vi "Read Status Byte Query.vi"(0 "VISA resource name":refnum<visa-resource-name>, 11 "error in (no error)":errorcluster) -> (4 "VISA resource name out":refnum<visa-resource-name>, 6 "Status Byte Register":T1, 15 "error out":errorcluster)   [LabVIEW 2018, in "XP Power PLS600.lvlib"]
doc: "Queries the <B>Status Byte</B>. Returns the decimal value of the binary-weighted sum of bits.\n\nEach bit represents a status in the instrument.\n\nBIT 0: Reserved\nBIT 1: Reserved\nBIT 2: Error in Queue\nBIT 3: QUES = Questionable Status Summary\nBIT 4: MAV = Message Available\nBIT 5: ESB = Event Status Byte Summary\nBIT 6: RQS = Request for Service\nBIT 7: OPER = Operation Event Summary"
uses:
  XP Power PLS600.lvlib
panel:
  # "BIT 0: Reserved\nBIT 1: Reserved\nBIT 2: Error in Queue\nBIT 3: QUES = Questionable Status Summary\nBIT 4: MAV = Message Available\nBIT 5: ESB = Event Status Byte Summary\nBIT 6: RQS = Request for Service\nBIT 7: OPER = Operation Event Summary"
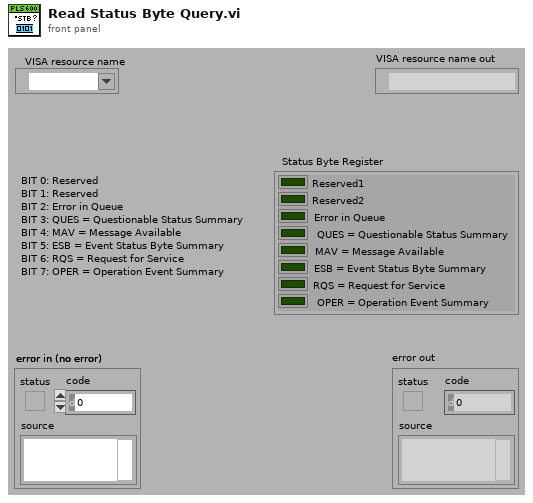
[diagram p1: front panel]
types:
  T1 = cluster{"Reserved1":bool, "Reserved2":bool, "Error in Queue":bool, "QUES = Questionable Status Summary":bool, "MAV = Message Available":bool, "ESB = Event Status Byte Summary":bool, "RQS = Request for Service":bool, "OPER = Operation Event Summary":bool}
  T2 = cluster{"Boolean array[0]":bool, "Boolean array[1]":bool, "Boolean array[2]":bool, "Boolean array[3]":bool, "Boolean array[4]":bool, "Boolean array[5]":bool, "Boolean array[6]":bool, "Boolean array[7]":bool}
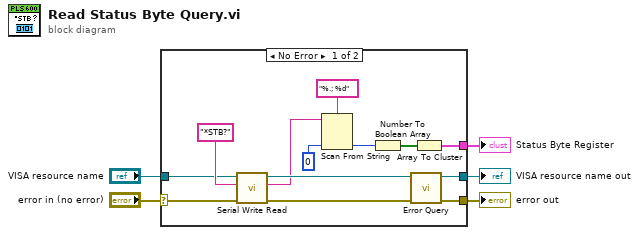
[diagram p0: block diagram]
diagram:
  n1 = case shown="No Error" "error in (no error)" {
    selector: "error in (no error)" -> [w13 w19]
    tunnel: [w18 _] -> w5
    tunnel: "VISA resource name" -> [w12 w20]
    tunnel: [w15 w20] -> w3
    tunnel: [w16 w19] -> w2
    frame No Error {
      n2 = call "Serial Write Read.vi"("error in (no error)"=w13, "Write Buffer"="*STB?" ("Command to Send (empty)"), "VISA resource name"=w12) -> ("error out"=w11:errorcluster, "Read Buffer"=w6:string, "VISA resource name out"=w10:refnum<visa-resource-name>)  [unwired: 6 in]
      n3 = Scan From String(format string="%.; %d" ("Format String"), input string=w6, default 1=u8 0 ("default value 1")) -> (output 1=w7:u8)  [unwired: 2 in, 3 out]
      n4 = Number To Boolean Array(number=w7) -> (Boolean array=w17:bool[])
      n5 = call "Error Query.vi"("error in (no error)"=w11, "VISA resource name"=w10) -> ("error out"=w16:errorcluster, "VISA resource name out"=w15:refnum<visa-resource-name>)  [unwired: 6 in, 2 out]
      n6 = Array To Cluster(array=w17) -> (cluster=w18:T2)
    }
    frame Error {
    }
  }
  "Status Byte Register" <- w5
  "VISA resource name out" <- w3
  "error out" <- w2
